vi "图像采集与保存-调用onnx模型.vi"(9 "Grab":bool, 11 "Camera Name":refnum<k21>="cam0" caption="IMAQdx Session") -> ()   [LabVIEW 2022 SP3]
doc: "The Grab and Attributes Setup example VI allows the user to view the current attributes and settings, update attribute settings, acquire images continuously, and display the images in an image control."
uses:
  <vilib>/vision/driver/IMAQdx.llb/IMAQdx Acquisition Mode.ctl
  <vilib>/vision/driver/IMAQdx.llb/IMAQdx Buffer Number Mode.ctl
  <vilib>/vision/driver/NI_Vision_Acquisition_Software.lvlib
panel:
  out "帧率/fps":dbl
  out "单张图片计算时间/ms":u32
  out "error out 2":errorcluster
  out "error out":errorcluster
  out "模型名":path
  out "return value":i32
  out "程序路径名":path
  out "Image out":T1(plugin-control)
  out "处理图片路径":path
  out "采集图片路径":path
  out "累计帧数":i32
  in  "采集帧间隔":i8
  in  "确定按钮":bool
  in  "Tab Control":T2(tab)
  in  "U32 Value Control":u32(slide) min=1 step=1 scale=1.0..4294967295.0
  in  "DBL Value Control":dbl(slide) min=2.2571161239684447 max=1000.0 step=1.0 scale=2.2571161239684447..1000.0
  in  "String Value Control":string
  in  "Enum Value Control":u32(ring) items=["Unicast", "Broadcast", "Multicast"]
  in  "Boolean Value Control":bool
  in  "Command Value Control":bool
  out "Tooltip":string="Gets/Sets the maximum number of outstanding events to queue."
  out "Units":string
  in  "Attribute Tree":string(tree)
  out "Frame Rate":dbl(knob) scale=0.0..100.0
  out "Image":T1(plugin-control)
  out "Buffer Number":u32
  in  "Stop":bool
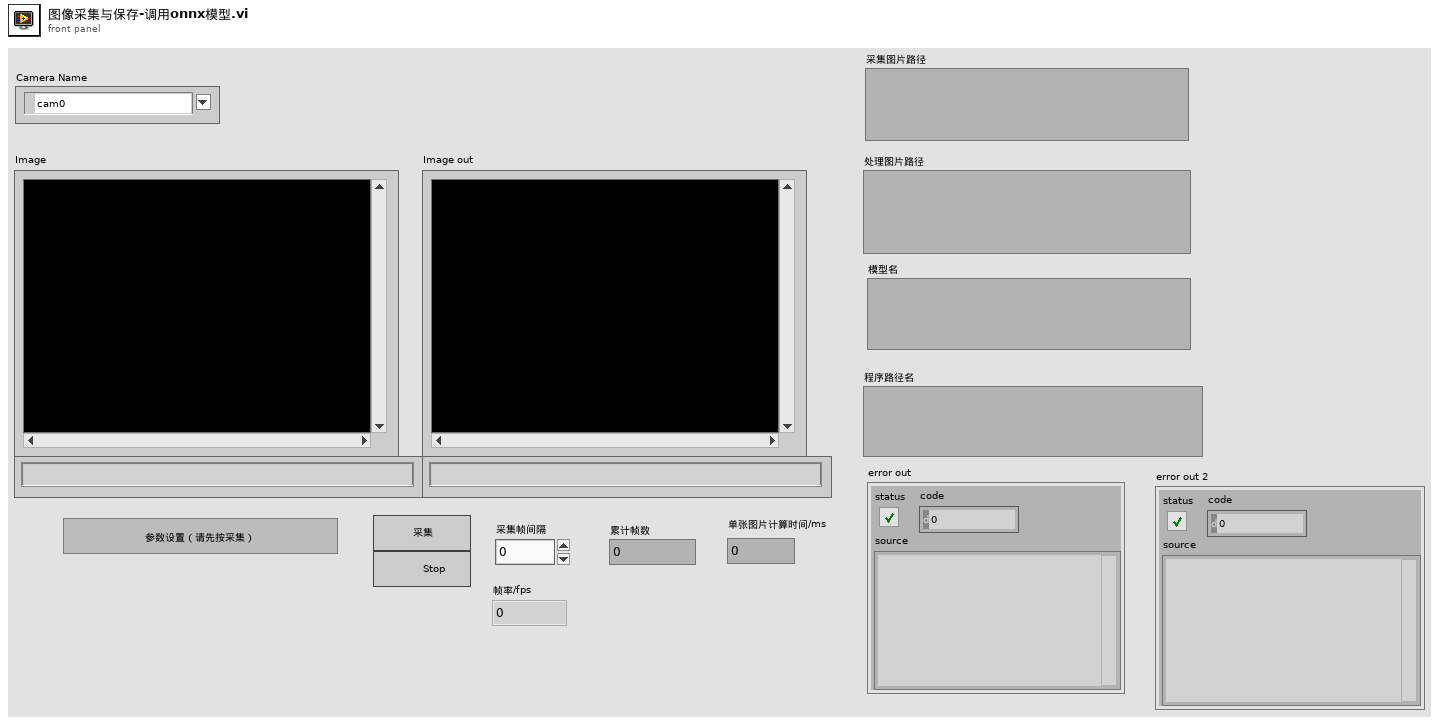
[diagram p1: front panel]
types:
  T1 = typedef "IMAQ Image.ctl" = refnum<image>
  T2 = enum32{"U32", "DBL", "String", "Enum", "Bool", "Command"}
  T3 = typedef "NI_Vision_Acquisition_Software.lvlib/IMAQdx Acquisition Mode.ctl" = enum32{"One Shot", "Continuous"}
  T4 = typedef "IMAQdx.ctl" = refnum<k21>
  T5 = cluster{"Tab Control":refnum<vi>, "U32 Value Control":refnum<vi>, "DBL Value Control":refnum<vi>, "String Value Control":refnum<vi>, "Enum Value Control":refnum<vi>, "Boolean Value Control":refnum<vi>, "Command Value Control":refnum<vi>}
  T6 = typedef "NI_Vision_Acquisition_Software.lvlib/IMAQdx Buffer Number Mode.ctl" = enum32{"Next", "Last", "Buffer Number", "Every", "Last New"}
  T7 = typedef "Image Type" = u32
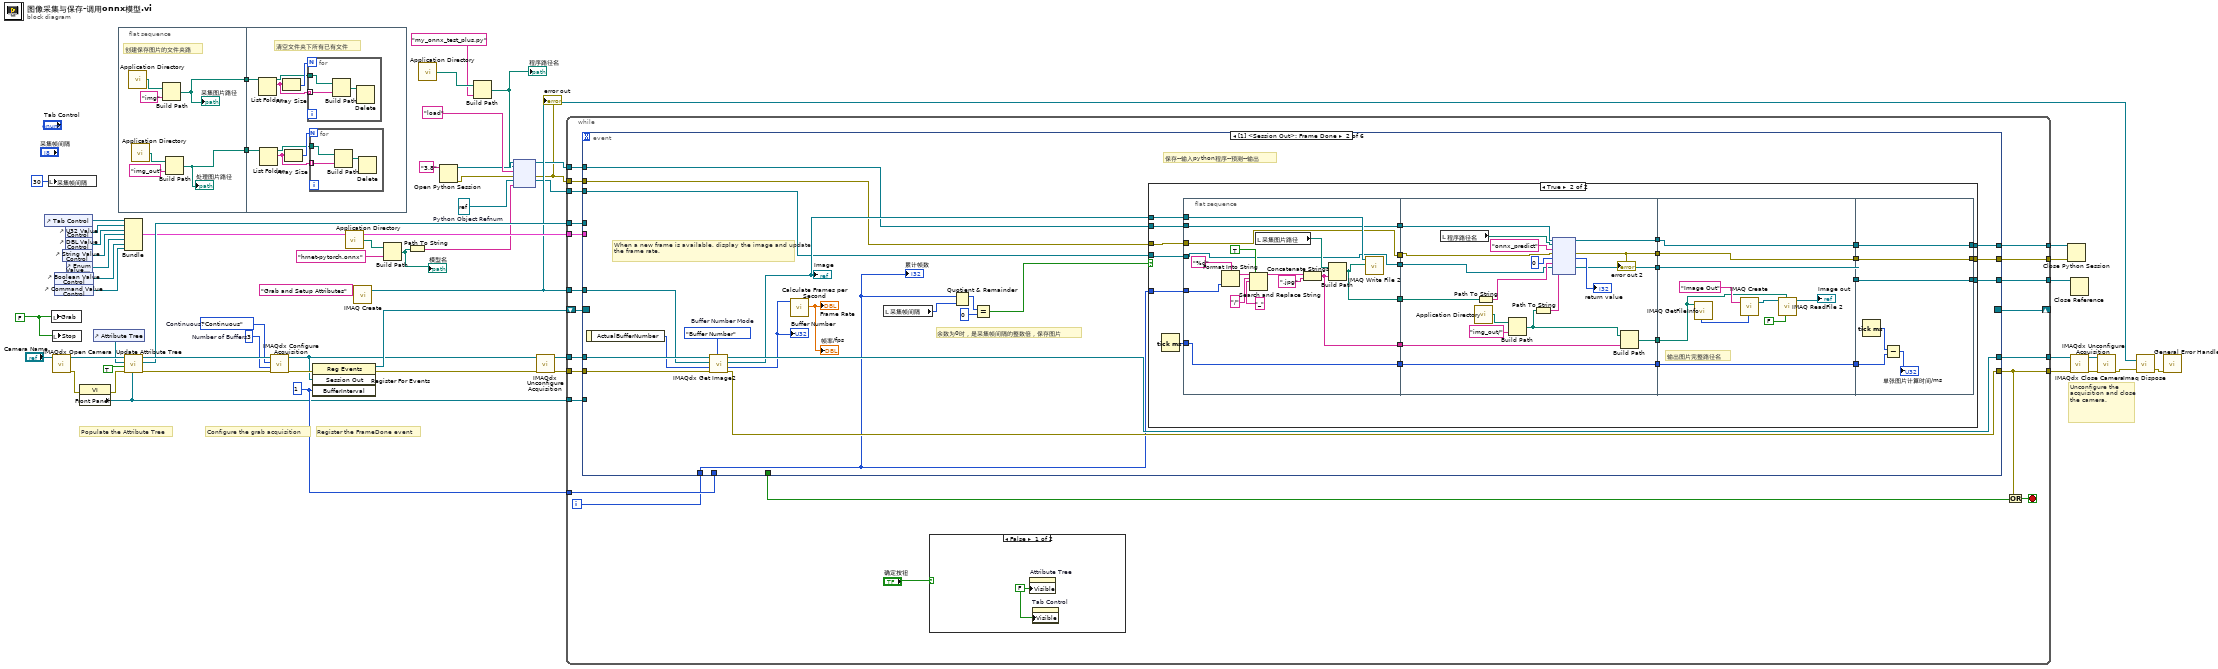
[diagram p0: block diagram]
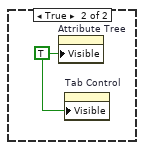
[diagram p2: hidden frame]
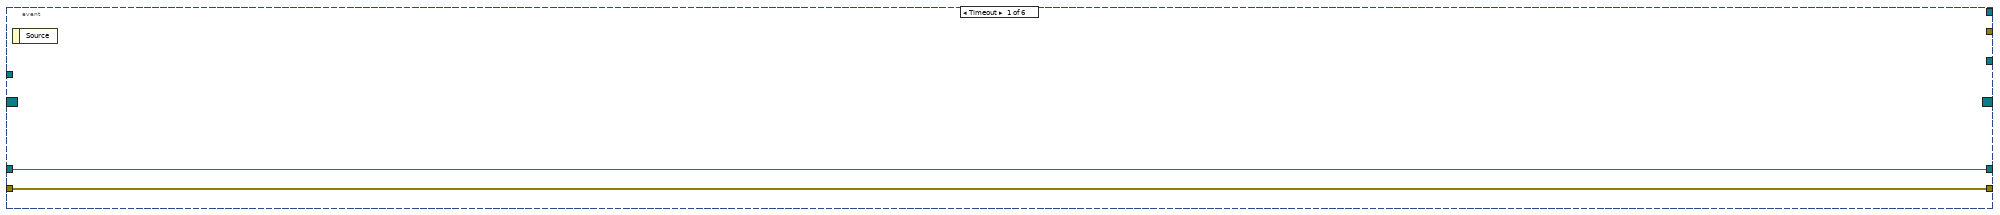
[diagram p3: hidden frame]
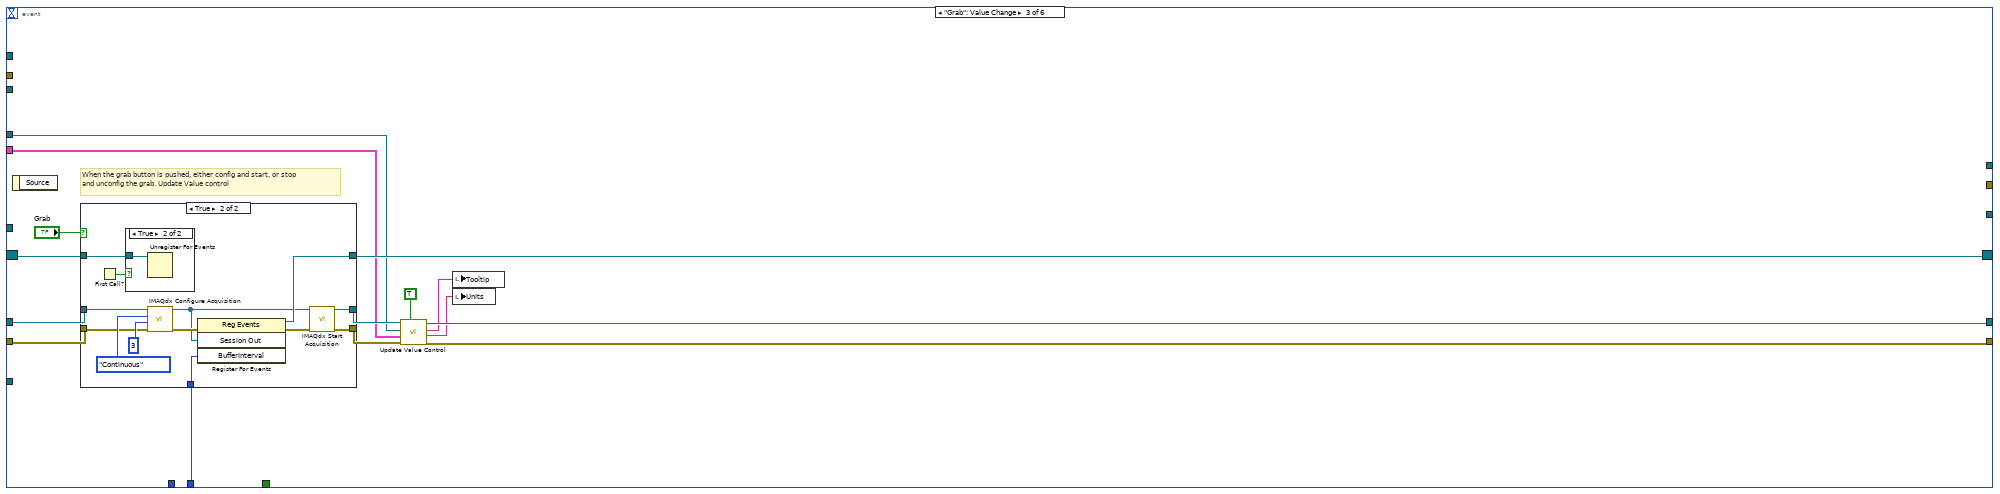
[diagram p5: hidden frame]
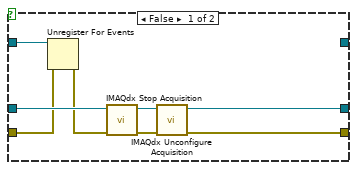
[diagram p6: hidden frame]
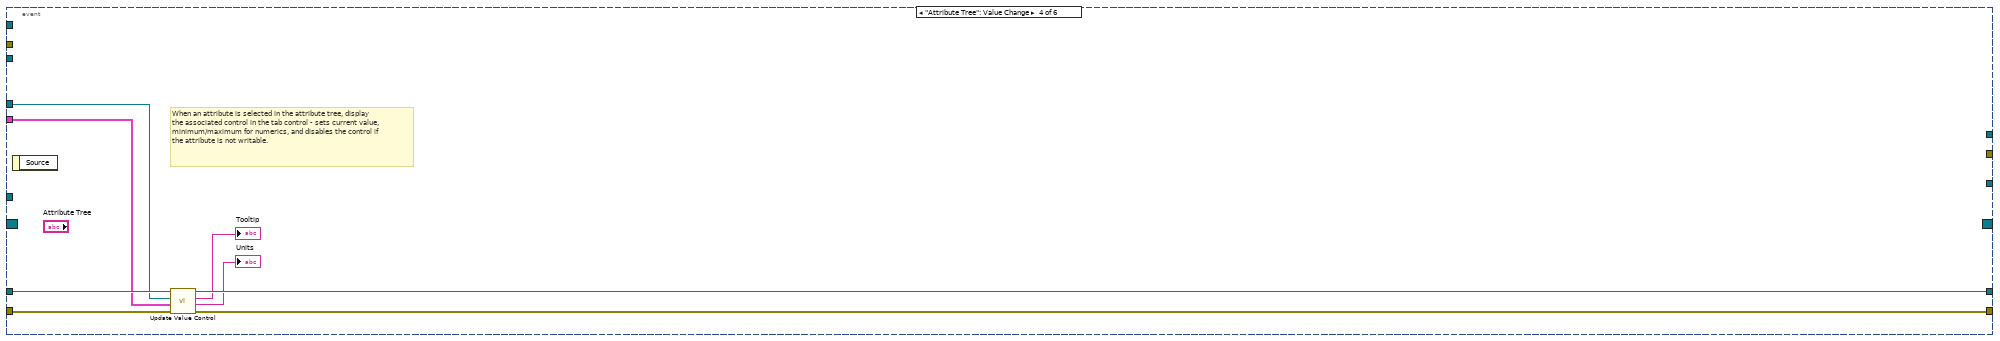
[diagram p8: hidden frame]
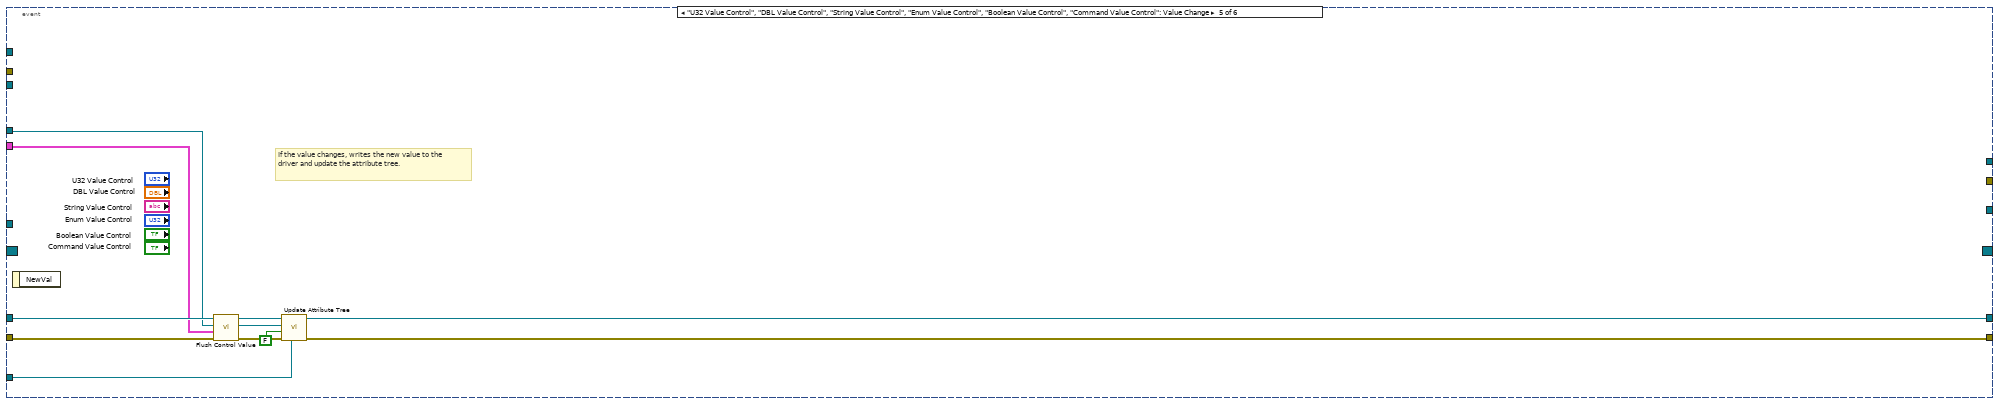
[diagram p9: hidden frame]
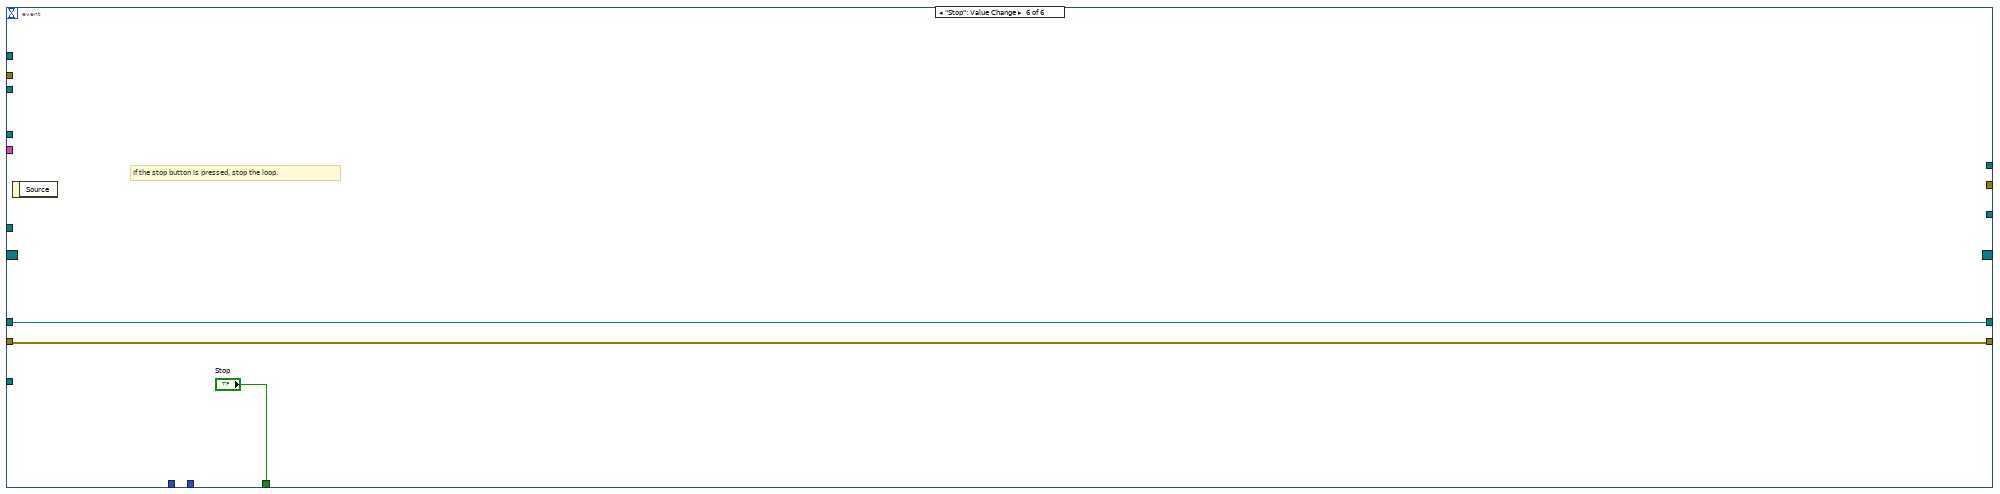
[diagram p10: hidden frame]
diagram:
  w10 = refnum<k38> refnum  # Python Object Refnum
  w1 = FALSE ("Grab")
  w38 = u32 1 ("BufferInterval")
  w24 = u32 3  # Number of Buffers
  w23 = IMAQdx_Acquisition_Mode."Continuous"  # Continuous?
  # "Unconfigure the acquisition and close the camera."
  # "Register the FrameDone event"
  # "Configure the grab acquisition"
  # "Populate the Attribute Tree"
  n1 = control-ref of="Tab Control"() -> (w28:refnum<vi>)
  n2 = local write "采集帧间隔"(i8 30 ("采集帧间隔")) -> ()
  n3 = local write "Grab"(w1) -> ()
  n4 = local write "Stop"(w1) -> ()
  n5 = call <vilib>:"IMAQdx Open Camera.vi"("Session In"="Camera Name") -> ("error out"=w41:errorcluster, "Session Out"=w46:T4)  [unwired: 2 in, 7 out]
  n6 = control-ref of="Boolean Value Control"() -> (w48:refnum<vi>)
  n7 = control-ref of="Command Value Control"() -> (w47:refnum<vi>)
  n8 = control-ref of="String Value Control"() -> (w52:refnum<vi>)
  n9 = control-ref of="U32 Value Control"() -> (w51:refnum<vi>)
  n10 = control-ref of="DBL Value Control"() -> (w50:refnum<vi>)
  n11 = control-ref of="Enum Value Control"() -> (w49:refnum<vi>)
  n12 = property class="VI"(error in=w41) -> (error out=w27:errorcluster, "Front Panel"=w25:refnum<vi>)  [unwired: 1 in, 1 out]
  n13 = control-ref of="Attribute Tree"() -> (w44:refnum<vi>)
  n14 = flat-sequence {
    tunnel: [w61] -> w21
    tunnel: [w58] -> w20
    tunnel: w21 -> [w68]
    tunnel: w20 -> [w64]
    frame #0 {
      # "创建保存图片的文件夹路"
      n15 = call <vilib>:"Application Directory.vi"() -> ("Application Directory"=w63:path)
      n16 = call <vilib>:"Application Directory.vi"() -> ("Application Directory"=w60:path)
      n17 = Build Path(base path=w63, name or relative path="img" ("名称或相对路径")) -> (appended path=w61:path)
      "采集图片路径" <- w61
      n18 = Build Path(base path=w60, name or relative path="img_out" ("名称或相对路径")) -> (appended path=w58:path)
      "处理图片路径" <- w58
    }
    frame #1 {
      # "清空文件夹下所有已有文件"
      n19 = List Folder(path=w68) -> (path out=w69:path, filenames=w71:string[])  [unwired: 3 in, 2 out]
      n20 = List Folder(path=w64) -> (path out=w65:path, filenames=w67:string[])  [unwired: 3 in, 2 out]
      n21 = Array Size(array=w71) -> (size(s)=w70:i32)
      n22 = Array Size(array=w67) -> (size(s)=w66:i32)
      n23 = for {
        N: w70 -> [_]
        tunnel: w69 -> [w76]
        tunnel: w71 -> [w75] mode=indexing
        n24 = Build Path(base path=w76, name or relative path=w75) -> (appended path=w77:path)
        n25 = Delete(path (use dialog)=w77) -> ()  [unwired: 4 in, 3 out]
      }
      n26 = for {
        N: w66 -> [_]
        tunnel: w65 -> [w73]
        tunnel: w67 -> [w72] mode=indexing
        n27 = Build Path(base path=w73, name or relative path=w72) -> (appended path=w74:path)
        n28 = Delete(path (use dialog)=w74) -> ()  [unwired: 4 in, 3 out]
      }
    }
  }
  n29 = Bundle("Tab Control"=w28, "U32 Value Control"=w51, "DBL Value Control"=w50, "String Value Control"=w52, "Enum Value Control"=w49, "Boolean Value Control"=w48, "Command Value Control"=w47) -> (w33:T5)  [unwired: 1 out]
  n30 = call "Update Attribute Tree.vi"("Panel Refnum In"=w25, "error in"=w27, "Flush Tree?"=TRUE, "Tree Control In"=w44, "Camera Name In"=w46) -> ("error out"=w26:errorcluster, "Tree Control Out"=w42:refnum<vi>, "Session Out"=w45:T4)  [unwired: 4 in]
  n31 = call <vilib>:"IMAQdx Configure Acquisition.vi"("error in"=w26, "Number of Buffers"=w24, "Continuous?"=w23, "Session In"=w45) -> ("error out"=w54:errorcluster, "Session Out"=w35:T4)  [unwired: 6 out]
  n32 = register-events(error in=w54, w35, w38) -> (reference out=w53:refnum<event-registration>, error out=w37:errorcluster)  [unwired: 1 in]
  n33 = call <vilib>:"Application Directory.vi"() -> ("Application Directory"=w7:path)
  n34 = call "IMAQ Create"("Image Name"="Grab and Setup Attributes") -> ("New Image"=w30:T1)  [unwired: 3 in, 2 out]
  n35 = Build Path(base path=w7, name or relative path="hrnet-pytorch.onnx") -> (appended path=w4:path)
  "模型名" <- w4
  n36 = Path To String(path=w4) -> (string=w5:string)
  n37 = call <vilib>:"Application Directory.vi"() -> ("Application Directory"=w14:path)
  n38 = Open Python Session(python version="3.8" ("Python版本")) -> (session out=w15:refnum<k35>, error out=w11:errorcluster)  [unwired: 2 in]
  n39 = Build Path(base path=w14, name or relative path="my_onnx_test_plus.py") -> (appended path=w12:path)
  "程序路径名" <- w12
  n40 = node(w15, w12, "load" ("function name"), w11, w10, w5) -> (w9:refnum<k35>, w8:errorcluster, w3:refnum<k38>)  [unwired: 1 in, 2 out]
  "error out" <- w8
  n41 = call <vilib>:"IMAQdx Unconfigure Acquisition.vi"("error in"=w37, "Session In"=w35) -> ("error out"=w36:errorcluster, "Session Out"=w34:T4)  [unwired: 8 out]
  n42 = while {
    tunnel: [w94] -> w40
    tunnel: w36 -> [w96]
    tunnel: w34 -> [w97]
    tunnel: [w87] -> w39
    tunnel: w30 -> [w95]
    tunnel: w42 -> [w92]
    tunnel: w25 -> [w91]
    tunnel: w38 -> [w89]
    shift-right: [w88] -> _
    shift-left: w53 -> [w93]
    tunnel: w33 -> [w86]
    tunnel: w9 -> [w83]
    tunnel: [w82] -> w18
    tunnel: [w81] -> w17
    tunnel: w8 -> [w80]
    tunnel: w3 -> [w79]
    tunnel: [w78] -> w2
    i -> [w85]
    stop <- w98 stop-if-true
    n43 = event shown="[1] <Session Out>: Frame Done" {
      selector: w93 -> [_ _ w212 _ _ _]
      dyn-events: [_ _ w214 _ _ _] -> w88
      timeout: _ -> [_ _ _ _ _ _]
      tunnel: w97 -> [w101 w123 w216 w246 w256 w258]
      tunnel: w96 -> [w102 w122 w211 w244 w257 w259]
      tunnel: w95 -> [_ w121 _ _ _ _]
      tunnel: [w101 w120 w204 w245 w252 w258] -> w94
      tunnel: [w102 w119 w208 w243 w248 w259] -> w87
      tunnel: w92 -> [_ _ w207 w241 w250 _]
      tunnel: w91 -> [_ _ _ _ w247 _]
      tunnel: [_ _ _ _ _ "Stop"] -> w90
      tunnel: w89 -> [_ _ w213 _ _ _]
      tunnel: w86 -> [_ _ w205 w242 w251 _]
      tunnel: w85 -> [_ w111 _ _ _ _]
      tunnel: w83 -> [_ w108 _ _ _ _]
      tunnel: [_ w107 _ _ _ _] -> w82
      tunnel: [_ w106 _ _ _ _] -> w81
      tunnel: w80 -> [_ w105 _ _ _ _]
      tunnel: w79 -> [_ w104 _ _ _ _]
      tunnel: [_ w103 _ _ _ _] -> w78
      event Timeout {
        n44 = event-data() -> ()  [unwired: 2 out]
      }
      event event #0x0 {
        w118 = IMAQdx_Buffer_Number_Mode."Buffer Number"  # Buffer Number Mode
        # "余数为0时，是采集帧间隔的整数倍，保存图片"
        # "保存--输入python程序--预测--输出"
        # "When a new frame is available, display the image and update the frame rate."
        n45 = event-data() -> ("ActualBufferNumber"=w117:u32)  [unwired: 1 out]
        n46 = call <vilib>:"IMAQdx Get Image2.vi"("Buffer Number Mode (Next)"=w118, "error in"=w122, "Buffer Number In"=w117, "Image In"=w121, "Session In"=w123) -> ("error out"=w119:errorcluster, "Buffer Number Out"=w116:u32, "Image Out"=w112:T1, "Session Out"=w120:T4)  [unwired: 3 in]
        "Image" <- w112
        "Buffer Number" <- w116
        n47 = call <vilib>:"Calculate Frames per Second.vi"("Buffer Number"=w116) -> ("Processed Frames/s"=→"Frame Rate" →"帧率/fps":dbl)  [unwired: 8 in, 2 out]
        n48 = local read "采集帧间隔"() -> (w110:i8)
        n49 = Quotient & Remainder(x=w111, y=w110) -> (x-y*floor(x/y)=w109:i32)  [unwired: 1 out]
        n50 = Equal?(x=w109, y=i8 0) -> (x = y?=w113:bool)
        n51 = case shown="True" w113 {
          tunnel: w111 -> [_ w150]
          tunnel: w112 -> [_ w149]
          tunnel: w108 -> [w126 w147]
          tunnel: [w126 w134] -> w107
          tunnel: [w125 w136] -> w106
          tunnel: w105 -> [w125 w145]
          tunnel: w104 -> [w124 w140]
          tunnel: [w124 w139] -> w103
          frame False {
          }
          frame True {
            n52 = Tick Count (ms)() -> (millisecond timer value=w127:u32)
            n53 = flat-sequence {
              tunnel: w150 -> [w159]
              tunnel: w149 -> [w158]
              tunnel: [w156] -> w148
              tunnel: w147 -> [w156]
              tunnel: [w155] -> w146
              tunnel: w145 -> [w154]
              tunnel: [w154] -> w144
              tunnel: [w153] -> w143
              tunnel: w140 -> [w152]
              tunnel: [w152] -> w141
              tunnel: [w151] -> w130
              tunnel: w127 -> [w151]
              tunnel: w148 -> [w177]
              tunnel: w146 -> [w185]
              tunnel: w144 -> [w175]
              tunnel: w143 -> [w181]
              tunnel: [w180] -> w142
              tunnel: w141 -> [w173]
              tunnel: [w171] -> w138
              tunnel: [w170] -> w137
              tunnel: [w169] -> w135
              tunnel: w130 -> [w167]
              tunnel: [w167] -> w129
              tunnel: w142 -> [w191]
              tunnel: w138 -> [w189]
              tunnel: w137 -> [w188]
              tunnel: w135 -> [w187]
              tunnel: [w189] -> w133
              tunnel: [w188] -> w132
              tunnel: [w187] -> w131
              tunnel: w129 -> [w186]
              tunnel: [w186] -> w128
              tunnel: [w199] -> w134
              tunnel: [w200] -> w136
              tunnel: [w201] -> w139
              tunnel: w133 -> [w201]
              tunnel: w132 -> [w200]
              tunnel: w131 -> [w199]
              tunnel: w128 -> [w197]
              frame #0 {
                n54 = Format Into String(format string="%d" ("Image Name"), w159) -> (resulting string=w160:string)  [unwired: 2 in, 1 out]
                n55 = Search and Replace String(replace all?=TRUE ("替换全部？(F)"), input string=w160, search string="/" ("搜索字符串"), replace string="_" ("替换字符串(\"\")")) -> (result string=w162:string)  [unwired: 4 in, 3 out]
                n56 = local read "采集图片路径"() -> (w157:path)
                n57 = Concatenate Strings(w162, ".jpg" ("字符串")) -> (w153:string)
                n58 = Build Path(base path=w157, name or relative path=w153) -> (appended path=w155:path)
                n59 = call-poly "IMAQ Write File 2"("File Path"=w155, "Image"=w158) -> ()  [unwired: 8 in, 2 out]
              }
              frame #1 {
                n60 = local read "程序路径名"() -> (w176:path)
                n61 = call <vilib>:"Application Directory.vi"() -> ("Application Directory"=w184:path)
                n62 = Path To String(path=w185) -> (string=w174:string)
                n63 = Build Path(base path=w184, name or relative path="img_out/" ("名称或相对路径")) -> (appended path=w182:path)
                n64 = Path To String(path=w182) -> (string=w168:string)
                n65 = node(w177, w176, "onnx_predict" ("function name"), w175, 0, w174, w173, w168) -> (w169:refnum<k35>, w170:errorcluster, →"return value":i32, w171:refnum<k38>)  [unwired: 2 in, 2 out]
                "error out 2" <- w170
                n66 = Build Path(base path=w182, name or relative path=w181) -> (appended path=w180:path)
              }
              frame #2 {
                # "输出图片完整路径名"
                n67 = call "IMAQ GetFileInfo"("File Path"=w191) -> ("Image Type"=w190:T7)  [unwired: 4 in, 6 out]
                n68 = call "IMAQ Create"("Image Name"="Image Out", "Image Type"=w190) -> ("New Image"=w193:T1)  [unwired: 3 in, 1 out]
                n69 = call "IMAQ ReadFile 2"("Use File Path Image Type"=FALSE, "File Path"=w191, "Image"=w193) -> ("Image Out"=→"Image out":T1)  [unwired: 4 in, 4 out]
              }
              frame #3 {
                n70 = Tick Count (ms)() -> (millisecond timer value=w198:u32)
                n71 = Subtract(x=w198, y=w197) -> (x-y=→"单张图片计算时间/ms":u32)
              }
            }
          }
        }
        "累计帧数" <- w111
      }
      event "Grab": Value Change {
        # "When the grab button is pushed, either config and start, or stop and unconfig the grab. Update Value control"
        n72 = event-data() -> ()  [unwired: 2 out]
        n73 = case shown="True" "Grab" {
          tunnel: w216 -> [w224 w235]
          tunnel: [w221 w237] -> w210
          tunnel: [w220 w236] -> w209
          tunnel: [_ w230] -> w214
          tunnel: w213 -> [_ w228]
          tunnel: w212 -> [w219 w226]
          tunnel: w211 -> [w217 w227]
          frame False {
            n74 = Unregister For Events(event registration refnum=w219, error in=w217) -> (error out=w218:errorcluster)
            n75 = call <vilib>:"IMAQdx Stop Acquisition.vi"("error in"=w218, "Session In"=w224) -> ("error out"=w222:errorcluster, "Session Out"=w223:T4)  [unwired: 8 out]
            n76 = call <vilib>:"IMAQdx Unconfigure Acquisition.vi"("error in"=w222, "Session In"=w223) -> ("error out"=w220:errorcluster, "Session Out"=w221:T4)  [unwired: 8 out]
          }
          frame True {
            n77 = First Call?() -> (First Call?: T/F=w225:bool)
            n78 = case shown="True" w225 {
              tunnel: w226 -> [_ w238]
              frame False {
              }
              frame True {
                n79 = Unregister For Events(event registration refnum=w238) -> ()  [unwired: 1 in, 1 out]
              }
            }
            n80 = call <vilib>:"IMAQdx Configure Acquisition.vi"("error in"=w227, "Number of Buffers"=u32 3, "Continuous?"=IMAQdx_Acquisition_Mode."Continuous", "Session In"=w235) -> ("error out"=w232:errorcluster, "Session Out"=w229:T4)  [unwired: 6 out]
            n81 = register-events(error in=w232, w229, w228) -> (reference out=w230:refnum<event-registration>, error out=w231:errorcluster)  [unwired: 1 in]
            n82 = call <vilib>:"IMAQdx Start Acquisition.vi"("error in"=w231, "Session In"=w229) -> ("error out"=w236:errorcluster, "Session Out"=w237:T4)  [unwired: 8 out]
          }
        }
        n83 = call "Update Value Control.vi"("Force update?"=TRUE, "error in (no error)"=w209, "Tab Control Ref In"=w205, "Tree Control In"=w207, "Session In"=w210) -> ("error out"=w208:errorcluster, "Units"=w202:string, "Tooltip"=w203:string, "Session Out"=w204:T4)  [unwired: 3 in]
        n84 = local write "Tooltip"(w203) -> ()
        n85 = local write "Units"(w202) -> ()
      }
      event "Attribute Tree": Value Change {
        # "When an attribute is selected in the attribute tree, display the associated control in the tab control - sets current value, minimum/maximum for numerics, and disables the control if the attribute is not writable."
        n86 = event-data() -> ()  [unwired: 2 out]
        n87 = call "Update Value Control.vi"("error in (no error)"=w244, "Tab Control Ref In"=w242, "Tree Control In"=w241, "Session In"=w246) -> ("error out"=w243:errorcluster, "Units"=→"Units":string, "Tooltip"=→"Tooltip":string, "Session Out"=w245:T4)  [unwired: 4 in]
      }
      event "U32 Value Control", "DBL Value Control", "String Value Control", "Enum Value Control", "Boolean Value Control", "Command Value Control": Value Change {
        # "If the value changes, writes the new value to the driver and update the attribute tree."
        n88 = event-data() -> ()  [unwired: 2 out]
        n89 = call "Flush Control Value.vi"("error in (no error)"=w257, "Tab Control Ref In"=w251, "Tree Control In"=w250, "Session In"=w256) -> ("error out"=w249:errorcluster, "Tree Control Out"=w254:refnum<vi>, "Session Out"=w255:T4)  [unwired: 5 in]
        n90 = call "Update Attribute Tree.vi"("Panel Refnum In"=w247, "error in"=w249, "Flush Tree?"=FALSE, "Tree Control In"=w254, "Camera Name In"=w255) -> ("error out"=w248:errorcluster, "Session Out"=w252:T4)  [unwired: 4 in, 1 out]
      }
      event "Stop": Value Change {
        # "If the stop button is pressed, stop the loop."
        n91 = event-data() -> ()  [unwired: 2 out]
      }
    }
    n92 = case shown="False" "确定按钮" {
      frame False {
        w99 = FALSE ("可见")
        n93 = property on="Attribute Tree" class="Tree (strict)"("Visible"=w99) -> ()  [unwired: 2 in, 2 out]
        n94 = property on="Tab Control" class="TabCtl (strict)"("Visible"=w99) -> ()  [unwired: 2 in, 2 out]
      }
      frame True {
        w100 = TRUE ("可见")
        n95 = property on="Attribute Tree" class="Tree (strict)"("Visible"=w100) -> ()  [unwired: 2 in, 2 out]
        n96 = property on="Tab Control" class="TabCtl (strict)"("Visible"=w100) -> ()  [unwired: 2 in, 2 out]
      }
    }
    n97 = Or(x=w87, y=w90) -> (x .or. y?=w98:bool)
  }
  n98 = Close Python Session(session in=w18, error in=w17) -> ()  [unwired: 1 out]
  n99 = Close Reference(reference=w2) -> ()  [unwired: 1 in, 1 out]
  n100 = call <vilib>:"IMAQdx Unconfigure Acquisition.vi"("error in"=w39, "Session In"=w40) -> ("error out"=w56:errorcluster, "Session Out"=w55:T4)  [unwired: 8 out]
  n101 = call <vilib>:"IMAQdx Close Camera.vi"("error in"=w56, "Session In"=w55) -> ("error out"=w32:errorcluster)  [unwired: 9 out]
  n102 = call "Imaq Dispose"("Image"=w30, "error in (no error)"=w32) -> ("error out"=w31:errorcluster)  [unwired: 4 in]
  n103 = call <vilib>:"General Error Handler.vi"("error in (no error)"=w31) -> ()  [unwired: 2 in, 13 out]
